vi "Tiempos.vi"() -> (3 "String":string)   [LabVIEW 2025]
panel:
  in  "stop":bool
  out "Boolean 3":bool
  in  "Dial 3":dbl(knob) scale=0.0..10.0
  out "Boolean 2":bool
  in  "Dial":dbl(knob) scale=0.0..10.0
  out "Boolean":bool
  out "Numeric":dbl
  # "Tiempo de mezclado"
  # "Tiempo de pesaje"
  # "Tiempo de reposo"
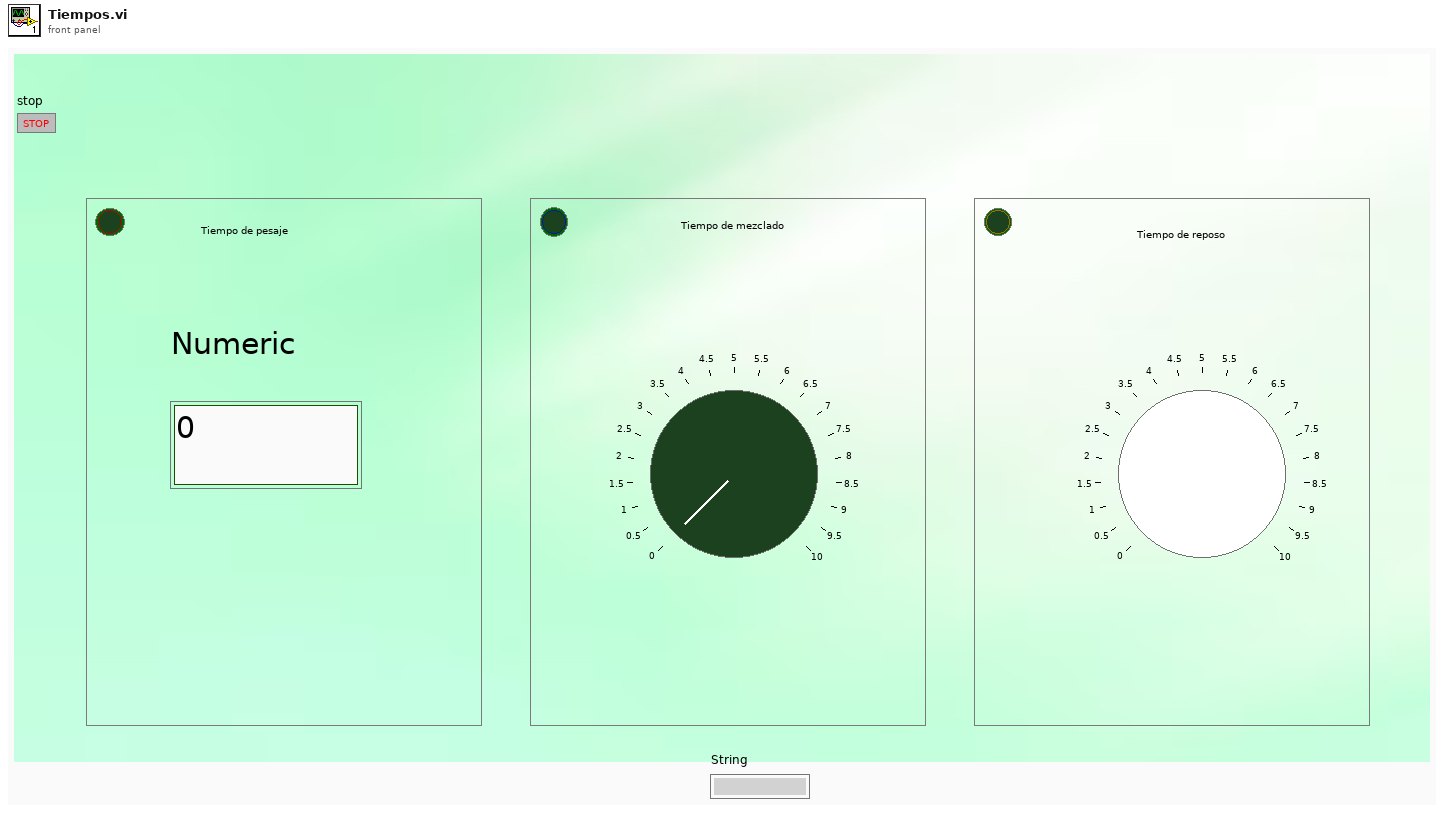
[diagram p1: front panel]
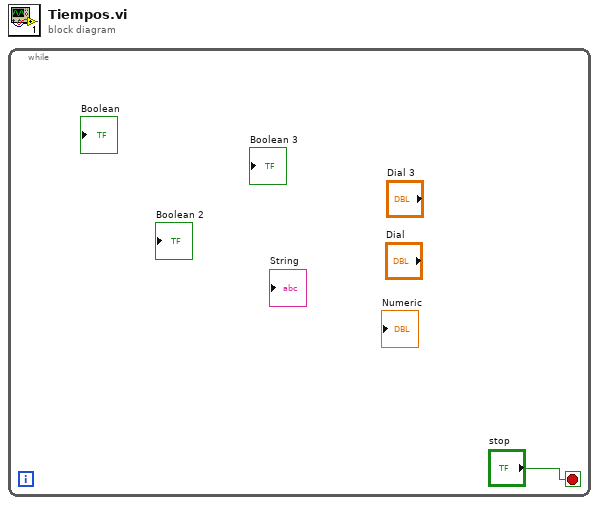
[diagram p0: block diagram]
diagram:
  n1 = while {
    stop <- "stop" stop-if-true
  }
